vi "3D-AlarmHistoryMessage.vi"(9 "Duration":string, 10 "Category":string(combo), 11 "Code":string) -> (3 "AlarmMessage":string[](array[string]))   [LabVIEW 2017]
panel:
  out "Time":string
  out "Date":string
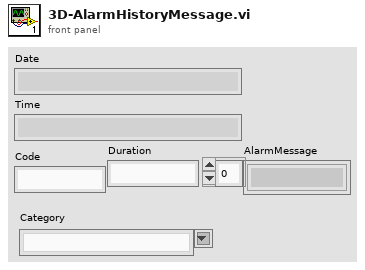
[diagram p1: front panel]
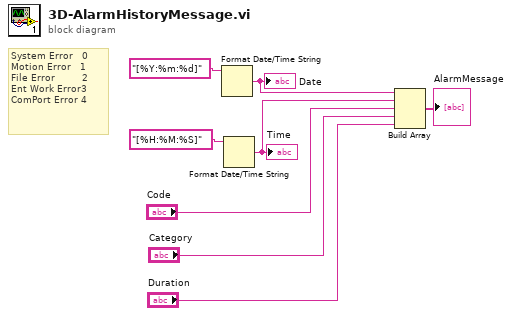
[diagram p0: block diagram]
diagram:
  # "System Error   0\nMotion Error   1\nFile Error         2\nEnt Work Error3\nComPort Error 4"
  n1 = Format Date/Time String(time format string (%c)="[%Y:%m:%d]" ("时间格式字符串(%c)")) -> (date/time string=w6:string)  [unwired: 2 in]
  "Date" <- w6
  n2 = Format Date/Time String(time format string (%c)="[%H:%M:%S]" ("时间格式字符串(%c)")) -> (date/time string=w5:string)  [unwired: 2 in]
  "Time" <- w5
  n3 = Build Array(w6, w5, "Code", "Category", "Duration") -> (→"AlarmMessage":string[])
